vi "Write Waveform to Buffer (DBL).vi"(8 "error in (no error)":errorcluster, 9 "Waveform Info":T1, 10 "Data":dbl[](array[numeric]), 11 "Waveform Buffer in":refnum<class "Waveform Buffer.lvclass">) -> (0 "error out":errorcluster, 3 "Waveform Buffer out":refnum<class "Waveform Buffer.lvclass">)   [LabVIEW 2015, in "Waveform Buffer.lvclass"]
uses:
  Waveform Buffer.lvclass
  Waveform Receive/Wfm Info.ctl
  Waveform Buffer.lvclass/Waveform Buffer.ctl
  DBL Waveform Buffer/DBL Waveform Buffer.lvclass
  DBL Waveform Buffer/DBL Waveform Buffer.lvclass/DBL Waveform Buffer.ctl
  Get Current Buffer Index.vi
  Get Buffer Length.vi
  Shift Point by Samples.vi
  Waveform Receive/Waveform Receive.lvclass
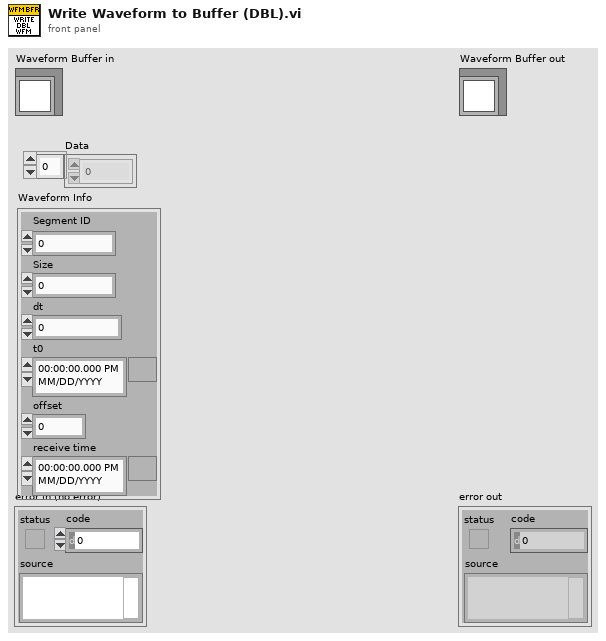
[diagram p1: front panel]
types:
  T1 = typedef "Waveform Receive.lvclass/Wfm Info.ctl" = cluster{"Segment ID":u64, "Size":i32, "dt":dbl, "t0":timestamp, "offset":u64, "receive time":timestamp}
  T2 = typedef "Waveform Buffer.lvclass/Buffer Data Type.ctl" = enum16{"Double", "ComplexDouble"}
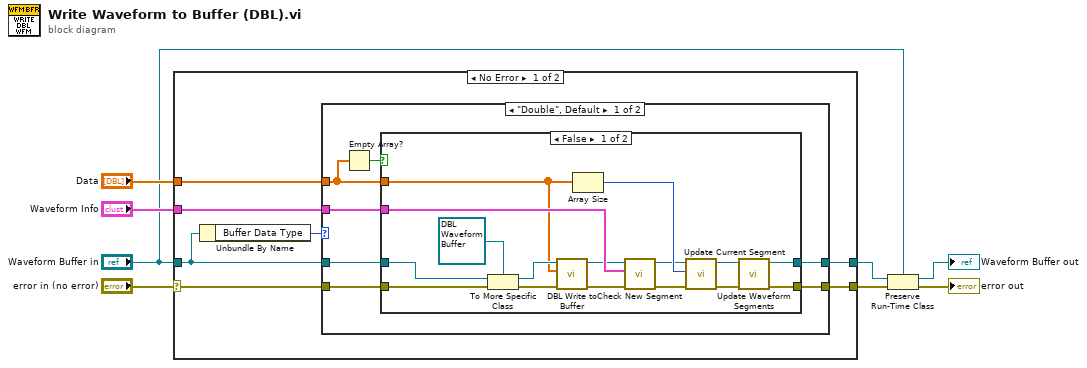
[diagram p0: block diagram]
diagram:
  n1 = case shown="No Error" "error in (no error)" {
    selector: "error in (no error)" -> [w13 w44]
    tunnel: [w9 w44] -> w4
    tunnel: [w10 w43] -> w5
    tunnel: "Waveform Buffer in" -> [w12 w43]
    tunnel: "Waveform Info" -> [w14 _]
    tunnel: "Data" -> [w15 _]
    frame No Error {
      n2 = Unbundle By Name(w12) -> ("Buffer Data Type"=w11:T2)
      n3 = case shown="\"Double\", Default" w11 {
        tunnel: w15 -> [w17 _]
        tunnel: w14 -> [w22 _]
        tunnel: w13 -> [w21 w41]
        tunnel: w12 -> [w20 w42]
        tunnel: [w18 w42] -> w10
        tunnel: [w19 w41] -> w9
        frame "Double", Default {
          n4 = Empty Array?(array=w17) -> (empty?=w16:bool)
          n5 = case shown="False" w16 {
            tunnel: w22 -> [w34 _]
            tunnel: w21 -> [w31 w39]
            tunnel: w20 -> [w30 w40]
            tunnel: w17 -> [w29 _]
            tunnel: [w24 w39] -> w19
            tunnel: [w23 w40] -> w18
            frame False {
              n6 = To More Specific Class(target class=refnum<class "DBL Waveform Buffer.lvclass"> refnum ("Waveform Data Logger Engine.lvlib:DBL Waveform Buffer.lvclass"), reference=w30, error in=w31) -> (specific class reference=w37:refnum<class "DBL Waveform Buffer.lvclass">, error out=w36:errorcluster)
              n7 = call "DBL Write to Buffer.vi"("error in (no error)"=w36, "Data"=w29, "DBL Waveform Buffer in"=w37) -> ("error out"=w27:errorcluster, "DBL Waveform Buffer out"=w28:refnum<class "DBL Waveform Buffer.lvclass">)  [unwired: 7 in]
              n8 = Array Size(array=w29) -> (size(s)=w35:i32)
              n9 = call "Check New Segment.vi"("error in (no error)"=w27, "Waveform Info"=w34, "Waveform Buffer in"=w28) -> ("error out"=w33:errorcluster, "Waveform Buffer out"=w32:refnum<class "DBL Waveform Buffer.lvclass">)  [unwired: 7 in]
              n10 = call "Update Current Segment.vi"("error in (no error)"=w33, "Waveform Size"=w35, "Waveform Buffer in"=w32) -> ("error out"=w25:errorcluster, "Waveform Buffer out"=w26:refnum<class "DBL Waveform Buffer.lvclass">)  [unwired: 7 in]
              n11 = call "Update Waveform Segments.vi"("error in (no error)"=w25, "Waveform Buffer in"=w26) -> ("error out"=w24:errorcluster, "Waveform Buffer out"=w23:refnum<class "DBL Waveform Buffer.lvclass">)  [unwired: 8 in]
            }
            frame True {
            }
          }
        }
        frame "ComplexDouble" {
        }
      }
    }
    frame Error {
    }
  }
  n12 = Preserve Run-Time Class(object in=w5, error in=w4, 2:"Waveform Buffer in") -> (object out=→"Waveform Buffer out":refnum<class "Waveform Buffer.lvclass">, error out=→"error out":errorcluster)
